vi "DebugWait.vi"   [LabVIEW 2010]
doc: "Adds a delay when running the code on the FPGA Emulator"
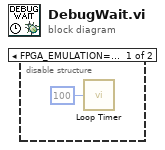
[diagram p0: block diagram]
diagram:
  n1 = disable-structure shown="FPGA_EMULATION==TRUE, default" {
    frame condition #0 {
      n2 = call "Loop Timer"("Count(mSec)"=u32 100) -> ()  [unwired: 1 out]
    }
    frame condition #1 (active) {
    }
  }
